vi "SetForceTrigger.vi"(8 "error in (no error)":errorcluster, 10 "body":T2, 11 "config in":T1) -> (0 "error out":errorcluster, 3 "config out":T1)   [LabVIEW 2017, in "Trigger.lvlib"]
uses:
  <vilib>/addons/InsightCM/Devices/Shared/Common/Trigger/Trigger.lvlib
  <vilib>/addons/InsightCM/MessageBus/MessageLibrary/Device/controls/DeviceForceTriggerRoutedMessageBody.ctl
  <vilib>/addons/InsightCM/Devices/Shared/Common/Trigger/controls/config.ctl
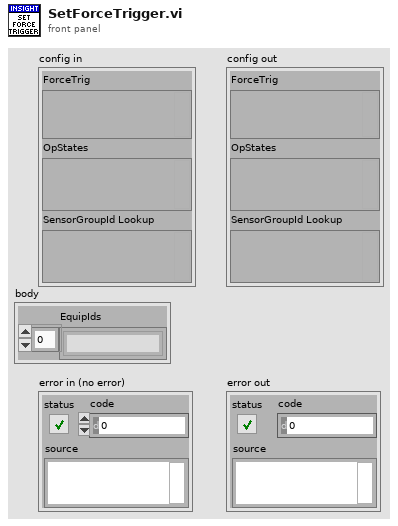
[diagram p1: front panel]
types:
  T1 = typedef "Trigger.lvlib/config.ctl" = cluster{"ForceTrig":variant, "OpStates":variant, "SensorGroupId Lookup":variant}
  T2 = typedef "DeviceForceTriggerRoutedMessageBody.ctl" = cluster{"EquipIds":string[]}
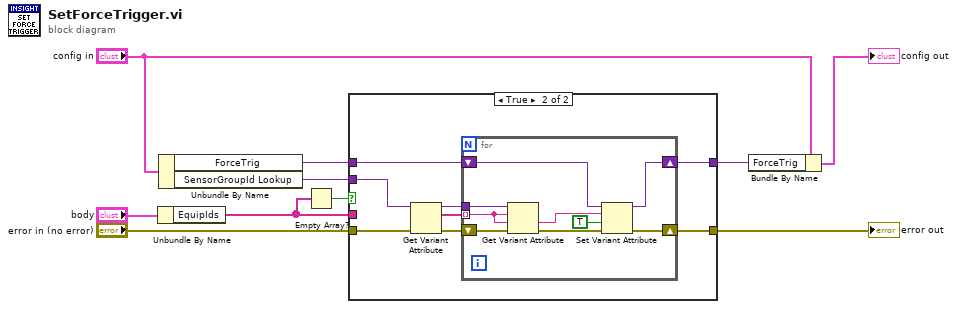
[diagram p0: block diagram]
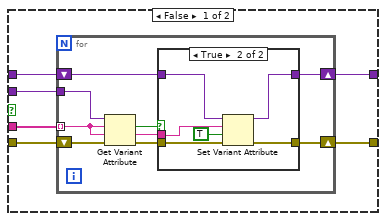
[diagram p2: hidden frame]
diagram:
  n1 = Unbundle By Name("body") -> ("EquipIds"=w1:string[])
  n2 = Unbundle By Name("config in") -> ("ForceTrig"=w5:variant, "SensorGroupId Lookup"=w6:variant)
  n3 = Empty Array?(array=w1) -> (empty?=w2:bool)
  n4 = case shown="True" w2 {
    tunnel: "error in (no error)" -> [w16 w41]
    tunnel: w1 -> [w15 _]
    tunnel: w6 -> [w14 w40]
    tunnel: w5 -> [w13 w36]
    tunnel: [w12 w35] -> w4
    tunnel: [w11 w34] -> w3
    frame False {
      n5 = for {
        shift-right: [w17] -> w11
        shift-left: w16 -> [w25]
        tunnel: w15 -> [w23] mode=indexing
        tunnel: w14 -> [w24]
        shift-right: [w18] -> w12
        shift-left: w13 -> [w19]
        n6 = Get Variant Attribute(Variant=w24, name=w23, default value (empty Variant)=w23, error in=w25) -> (found=w22:bool, value=w20:string, error out=w21:errorcluster)  [unwired: 1 out]
        n7 = case shown="True" w22 {
          tunnel: w21 -> [w26 w32]
          tunnel: w20 -> [_ w31]
          tunnel: w19 -> [w27 w33]
          tunnel: [w27 w29] -> w18
          tunnel: [w26 w28] -> w17
          frame False {
          }
          frame True {
            n8 = Set Variant Attribute(Variant=w33, name=w31, value=TRUE ("ForceTrigger"), error in=w32) -> (Variant out=w29:variant, error out=w28:errorcluster)  [unwired: 1 out]
          }
        }
      }
    }
    frame True {
      n9 = Get Variant Attribute(Variant=w40, error in=w41) -> (duplicate Variant=w38:variant, names=w37:string[], error out=w39:errorcluster)  [unwired: 2 in, 1 out]
      n10 = for {
        shift-right: [w44] -> w34
        shift-left: w39 -> [w48]
        tunnel: w38 -> [w50]
        tunnel: w37 -> [w49] mode=indexing
        shift-right: [w43] -> w35
        shift-left: w36 -> [w46]
        n11 = Get Variant Attribute(Variant=w50, name=w49, default value (empty Variant)=w49, error in=w48) -> (value=w42:string, error out=w45:errorcluster)  [unwired: 2 out]
        n12 = Set Variant Attribute(Variant=w46, name=w42, value=TRUE ("ForceTrigger"), error in=w45) -> (Variant out=w43:variant, error out=w44:errorcluster)  [unwired: 1 out]
      }
    }
  }
  "error out" <- w3
  n13 = Bundle By Name(cluster="config in", "ForceTrig"=w4) -> (→"config out":T1)
